vi "计时显示.vi"(10 "数值":i32) -> (1 "Cluster":T1 caption="簇", 2 "Cluster 2":T1 caption="簇")   [LabVIEW 2024]
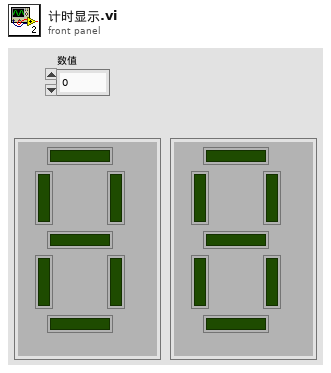
[diagram p1: front panel]
types:
  T1 = cluster{"布尔":bool, "布尔 5":bool, "布尔 4":bool, "布尔 2":bool, "布尔 6":bool, "布尔 7":bool, "布尔 3":bool}
  T2 = cluster{"布尔 7":bool, "布尔 2":bool, "布尔 3":bool, "布尔 4":bool, "布尔 6":bool, "布尔 5":bool, "布尔":bool}
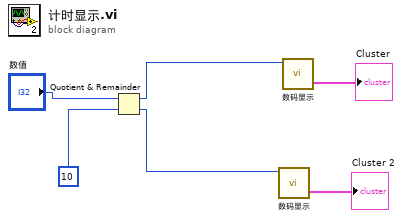
[diagram p0: block diagram]
diagram:
  n1 = Quotient & Remainder(x="数值", y=10) -> (x-y*floor(x/y)=w4:i32, floor(x/y)=w1:i32)
  n2 = call "数码显示.vi"("数值"=w1) -> ("Cluster"=→"Cluster 2":T2)  [unwired: 10 in]
  n3 = call "数码显示.vi"("数值"=w4) -> ("Cluster"=→"Cluster":T2)  [unwired: 10 in]
